vi "Simulador RLC v2.vi"() -> ()   [LabVIEW 2020]
uses:
  <vilib>/Utility/file.llb/Read Delimited Spreadsheet (DBL).vi
  <vilib>/measure/NI_MABase.lvlib
panel:
  out "Delta T da Onda\nEscolhida":dbl
  in  "Arquivo texto da onda":path
  out "ONDA DE ENTRADA e \nVOLTAGEM NO CAPACITOR":dbl[][](graph)
  out "ONDA DE ENTRADA e CORRENTE":dbl[][](graph)
  in  "?":T1={"Taxa de Amostragem"=1000.0, "Número de amostras"=1} {"Número de amostras" min=1 scale=1.0..20000.0; "Taxa de Amostragem" format="%#.6g"}
  in  "C - Capacitância":dbl
  in  "L -  Indutância":dbl
  in  "?":i32(knob) scale=0.0..2.0
  in  "R - Resistência":dbl
  in  "Amplitude":dbl
  in  "Duty Cicle":dbl
  in  "Frequência":dbl
  # "SIMULADOR RLC"
  # "Onda Senoidal"
  # "Onda Quadrada"
  # "Onda de um Arquivo"
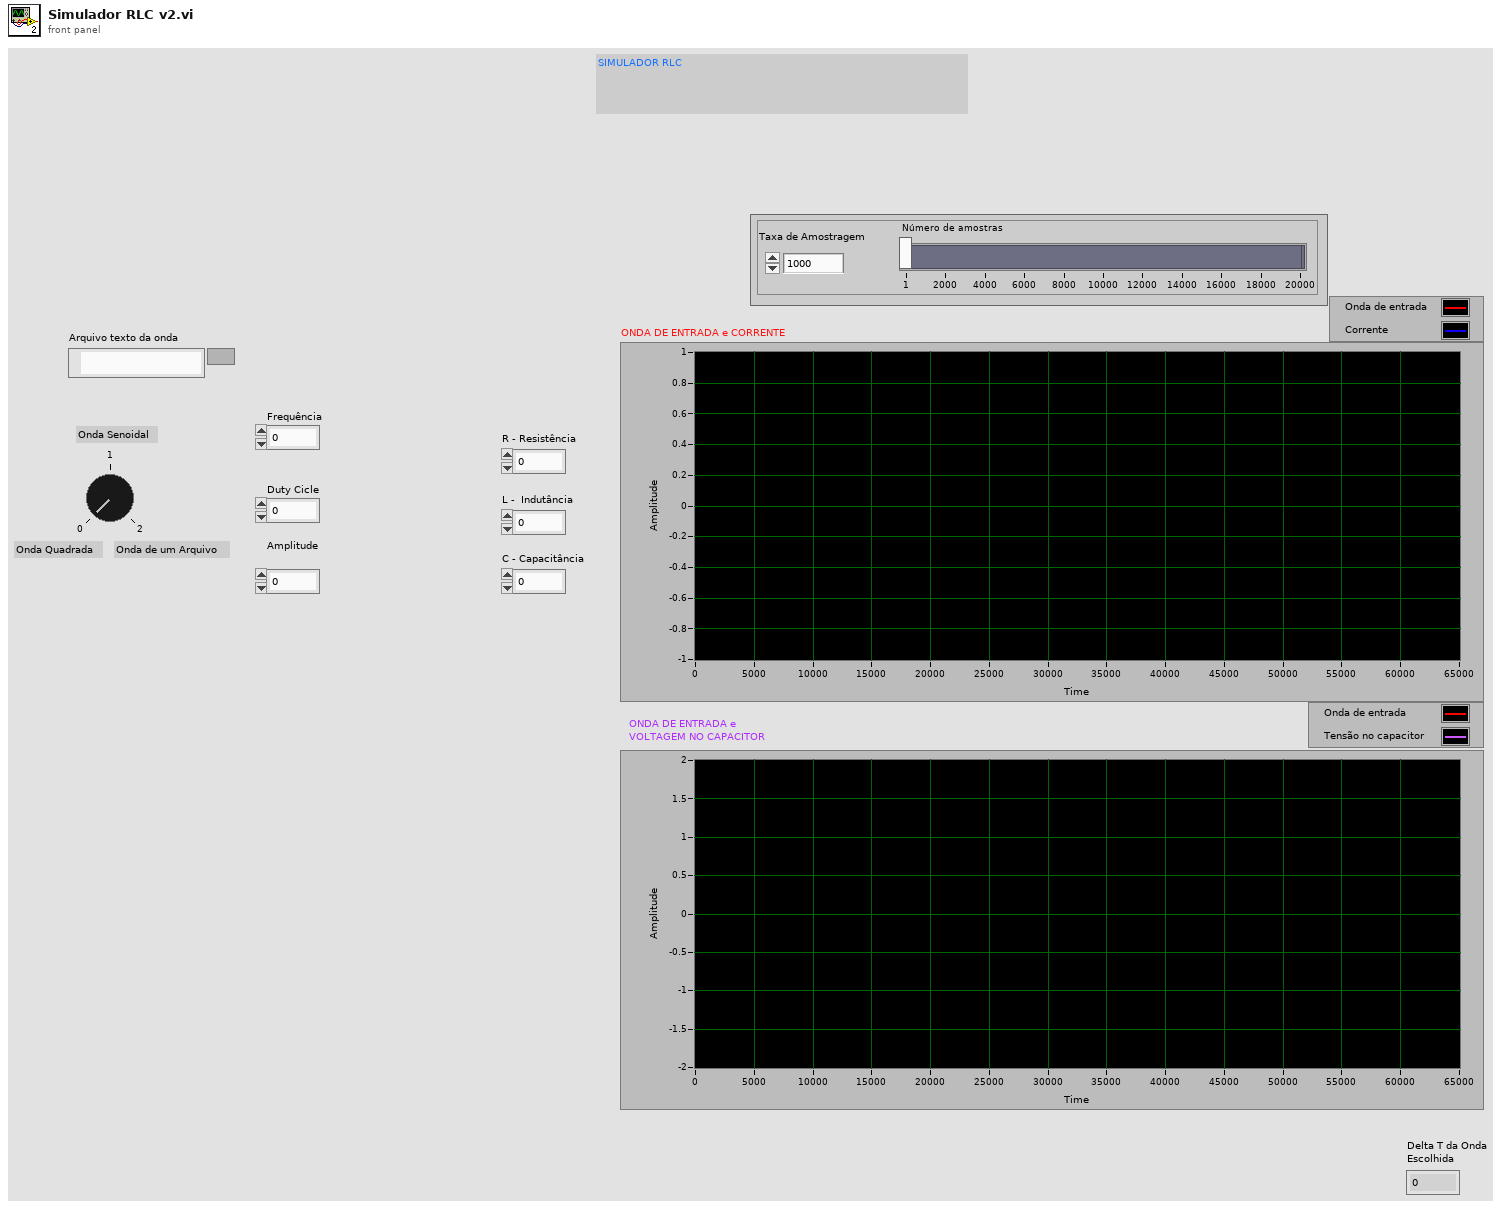
[diagram p1: front panel]
types:
  T1 = cluster{"Taxa de Amostragem":dbl, "Número de amostras":u32}
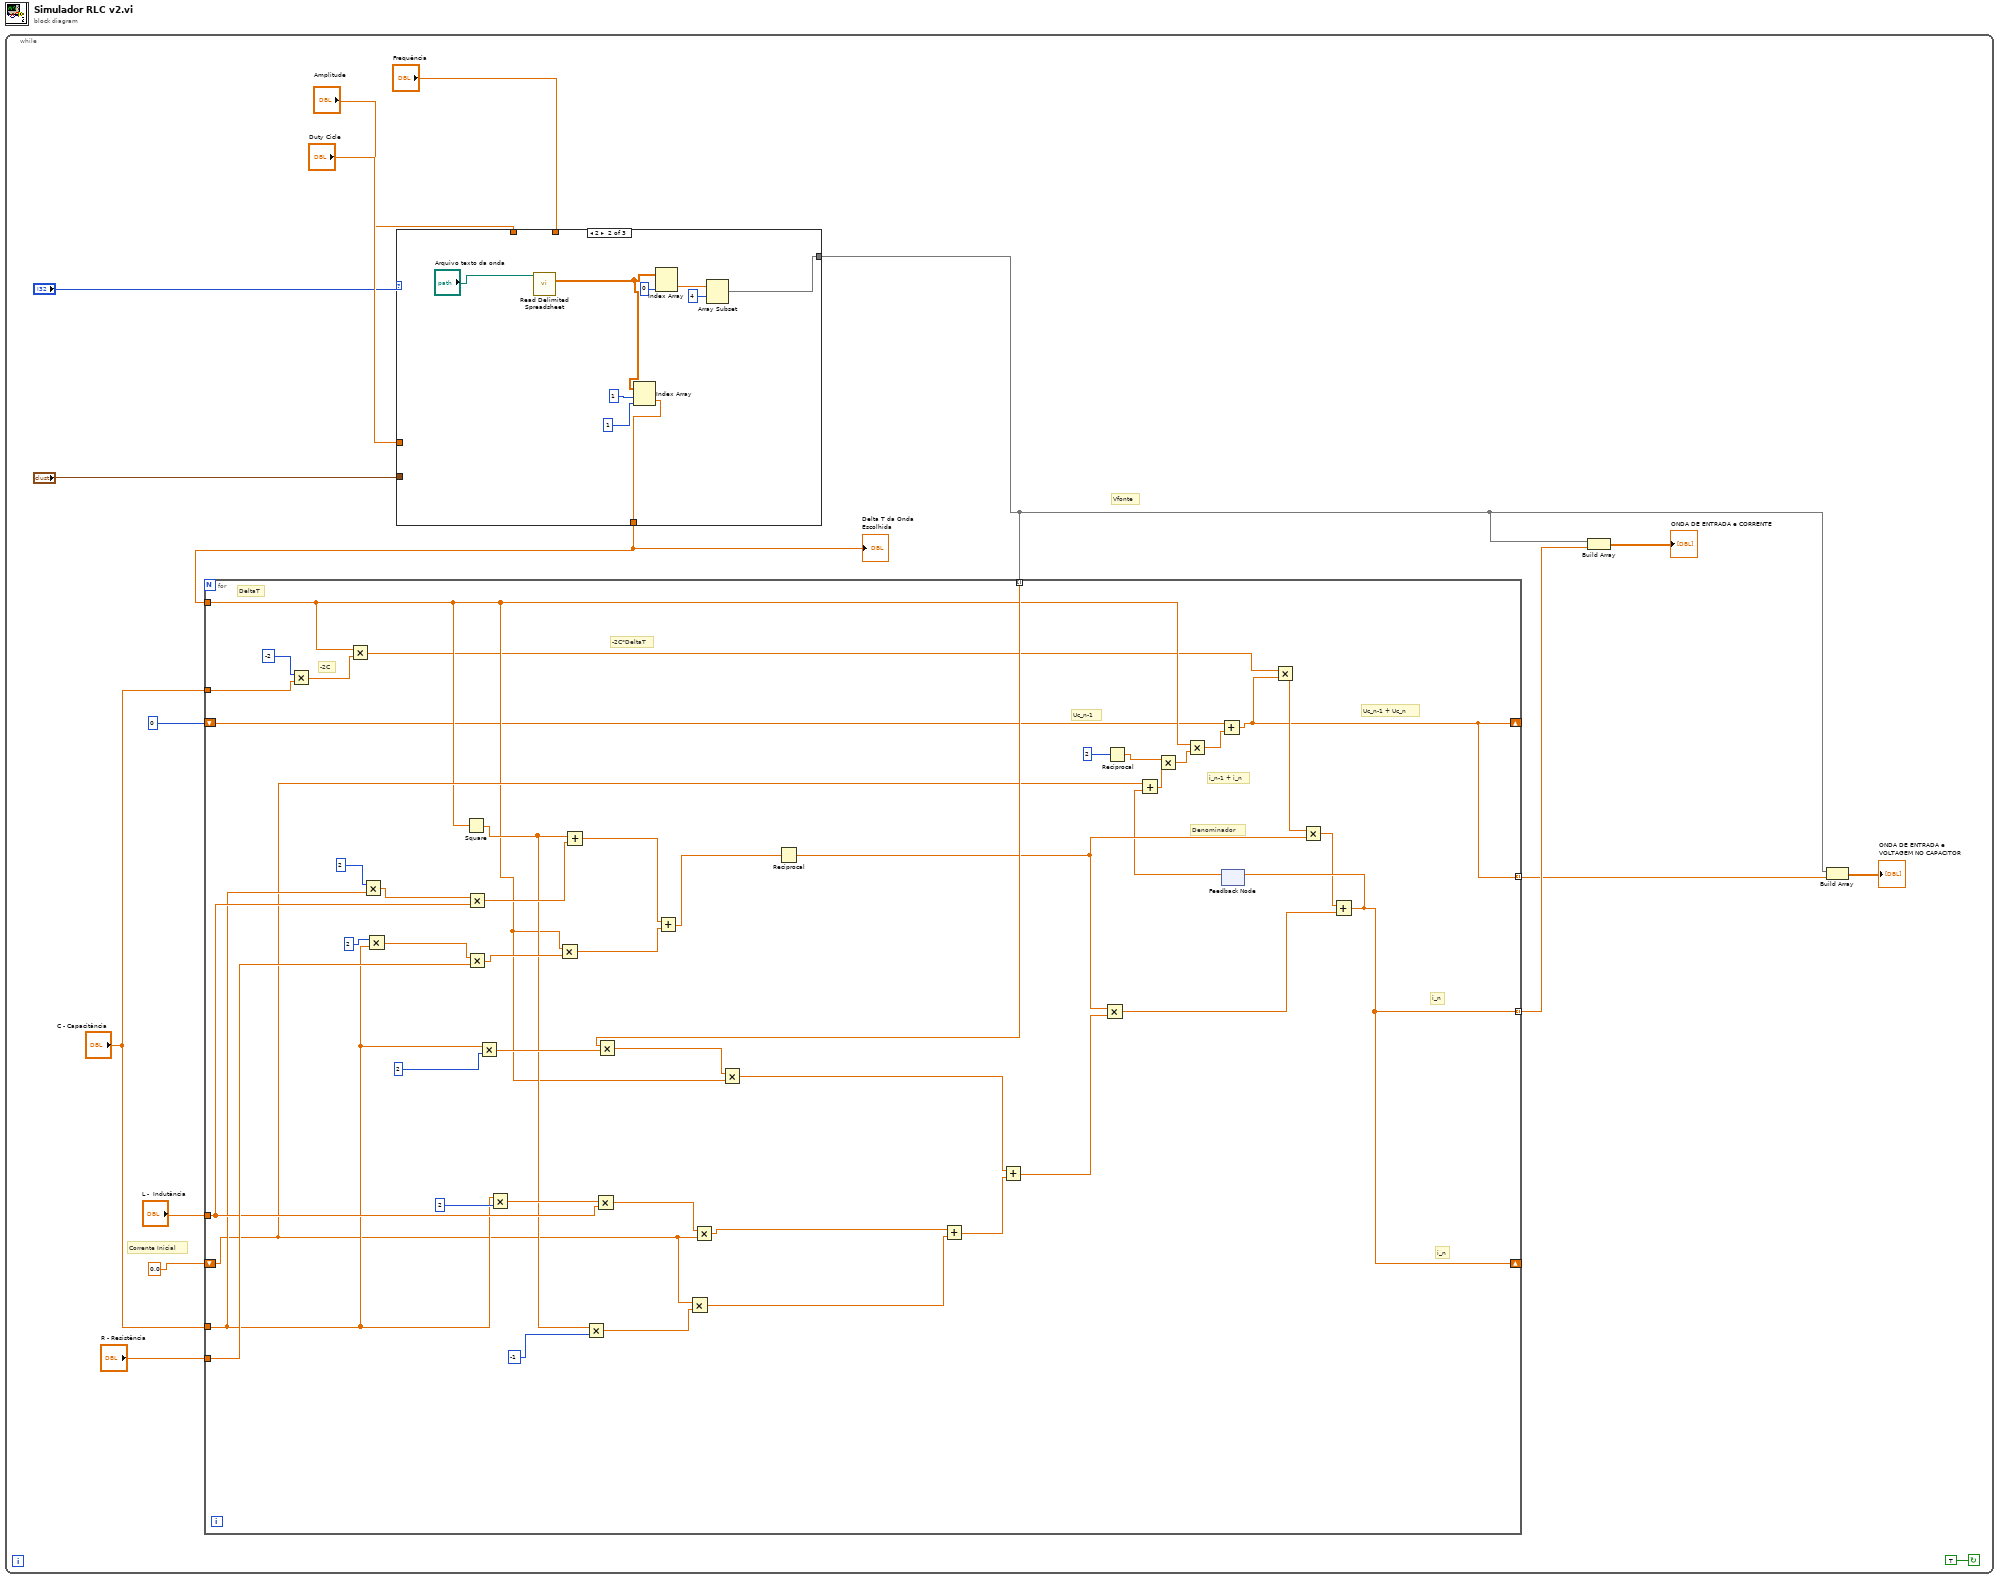
[diagram p0: block diagram]
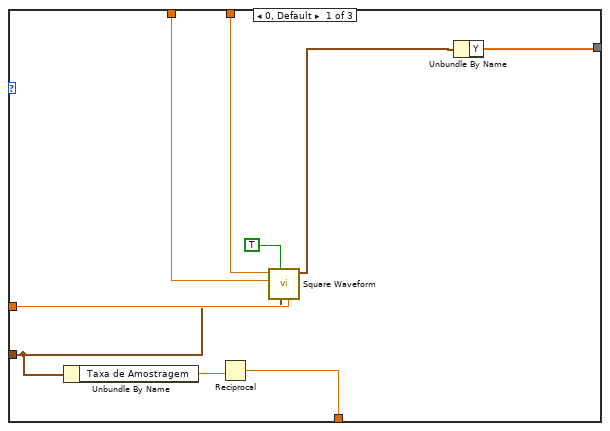
[diagram p2: hidden frame]
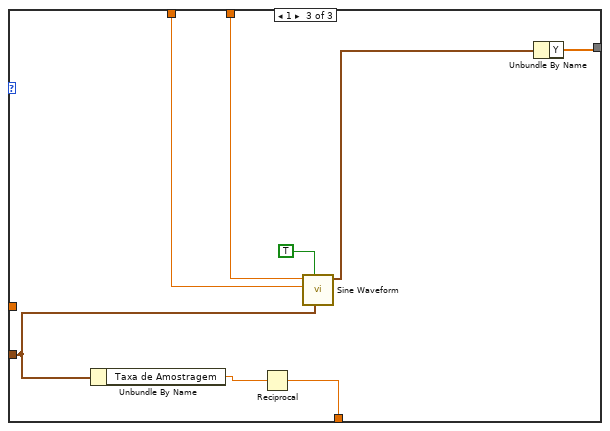
[diagram p3: hidden frame]
diagram:
  n1 = while {
    stop <- TRUE continue-if-true
    # "Vfonte"
    # "Corrente Inicial"
    n2 = case shown="2" "?" {
      tunnel: "Amplitude" -> [w72 _ w88]
      tunnel: "Frequência" -> [w71 _ w89]
      tunnel: "Duty Cicle" -> [w70 _ _]
      tunnel: [w67 w78 w85] -> w3
      tunnel: "?" -> [w65 _ w84]
      tunnel: [w64 w74 w82] -> w1
      frame 0, Default {
        n3 = Unbundle By Name(w65) -> ("Taxa de Amostragem"=w66:dbl)
        n4 = Reciprocal(x=w66) -> (1/x=w64:dbl)
        n5 = call <vilib>:"Square Waveform.vi"("duty cycle (%)"=w70, "sampling info"=w65, "reset signal"=TRUE, "amplitude"=w72, "frequency"=w71) -> ("signal out"=w68:waveform(dbl))  [unwired: 5 in, 1 out]
        n6 = Unbundle By Name(w68) -> ("Y"=w67:dbl[])
      }
      frame 2 {
        n7 = call-poly <vilib>:"Read Delimited Spreadsheet.vi"("file path (dialog if empty)"="Arquivo texto da onda") -> ("all rows"=w76:dbl[][])  [unwired: 9 in, 5 out]
        n8 = Index Array(array=w76, index (row)=1 ("disabled index (col)"), index (col)=1 ("disabled index (col)")) -> (element=w74:dbl)
        n9 = Index Array(array=w76, index (col)=0 ("disabled index (col)")) -> (element=w79:dbl[])  [unwired: 1 in]
        n10 = Array Subset(array=w79, index=4) -> (w78:dbl[])  [unwired: 1 in]
      }
      frame 1 {
        n11 = Unbundle By Name(w84) -> ("Taxa de Amostragem"=w83:dbl)
        n12 = Reciprocal(x=w83) -> (1/x=w82:dbl)
        n13 = call <vilib>:"Sine Waveform.vi"("sampling info"=w84, "reset signal"=TRUE, "amplitude"=w88, "frequency"=w89) -> ("signal out"=w86:waveform(dbl))  [unwired: 6 in, 1 out]
        n14 = Unbundle By Name(w86) -> ("Y"=w85:dbl[])
      }
    }
    "Delta T da Onda\nEscolhida" <- w1
    n15 = for {
      tunnel: w3 -> [w54] mode=indexing
      tunnel: w1 -> [w28]
      tunnel: [w20] -> w7 mode=indexing
      shift-right: [w20] -> _
      shift-left: 0.0 -> [w33]
      tunnel: "R - Resistência" -> [w41]
      tunnel: "L -  Indutância" -> [w40]
      tunnel: "C - Capacitância" -> [w39]
      tunnel: "C - Capacitância" -> [w36]
      shift-right: [w18] -> _
      shift-left: 0 -> [w26]
      tunnel: [w18] -> w5 mode=indexing
      # "Uc_n-1"
      # "-2C*DeltaT"
      # "-2C"
      # "Denominador"
      # "DeltaT"
      # "i_n"
      # "i_n"
      # "Uc_n-1 + Uc_n"
      # "i_n-1 + i_n"
      n16 = Multiply(x=-2, y=w36) -> (x*y=w34:dbl)
      n17 = Multiply(x=w28, y=w34) -> (x*y=w25:dbl)
      n18 = Multiply(x=2, y=w39) -> (x*y=w62:dbl)
      n19 = Multiply(x=2, y=w39) -> (x*y=w59:dbl)
      n20 = Square(x=w28) -> (x^2=w37:dbl)
      n21 = Multiply(x=w62, y=w40) -> (x*y=w61:dbl)
      n22 = Multiply(x=w59, y=w41) -> (x*y=w58:dbl)
      n23 = Multiply(x=w39, y=2) -> (x*y=w53:dbl)
      n24 = Multiply(x=w39, y=2) -> (x*y=w50:dbl)
      n25 = Multiply(x=w28, y=w58) -> (x*y=w56:dbl)
      n26 = Add(x=w37, y=w61) -> (x+y=w57:dbl)
      n27 = Multiply(x=w37, y=-1) -> (x*y=w45:dbl)
      n28 = Multiply(x=w50, y=w40) -> (x*y=w44:dbl)
      n29 = Multiply(x=w54, y=w53) -> (x*y=w52:dbl)
      n30 = Add(x=w57, y=w56) -> (x+y=w47:dbl)
      n31 = Multiply(x=w33, y=w45) -> (x*y=w42:dbl)
      n32 = Multiply(x=w44, y=w33) -> (x*y=w43:dbl)
      n33 = Multiply(x=w52, y=w28) -> (x*y=w49:dbl)
      n34 = Reciprocal(x=w47) -> (1/x=w24:dbl)
      n35 = Add(x=w43, y=w42) -> (x+y=w48:dbl)
      n36 = Add(x=w49, y=w48) -> (x+y=w46:dbl)
      n37 = Multiply(x=w24, y=w46) -> (x*y=w22:dbl)
      n38 = Reciprocal(x=2) -> (1/x=w31:dbl)
      n39 = feedback #1() -> (w21:dbl)  [unwired: 1 in]
      n40 = Add(x=w33, y=w21) -> (x+y=w30:dbl)
      n41 = Multiply(x=w31, y=w30) -> (x*y=w29:dbl)
      n42 = Multiply(x=w28, y=w29) -> (x*y=w27:dbl)
      n43 = Add(x=w26, y=w27) -> (x+y=w18:dbl)
      n44 = Multiply(x=w25, y=w18) -> (x*y=w23:dbl)
      n45 = Multiply(x=w23, y=w24) -> (x*y=w19:dbl)
      n46 = Add(x=w19, y=w22) -> (x+y=w20:dbl)
      n47 = feedback-in #1(w20) -> ()
    }
    n48 = Build Array(w3, w7) -> (→"ONDA DE ENTRADA e CORRENTE":dbl[][])
    n49 = Build Array(w3, w5) -> (→"ONDA DE ENTRADA e \nVOLTAGEM NO CAPACITOR":dbl[][])
  }
